vi "Create_Error_log_folders.vi"(0 "Log Filename":string, 1 "Days ago":dbl, 2 "Log Folder":string, 3 "Per Day Log File?":bool) -> (5 "Local Log File":path, 7 "exists?":bool)   [LabVIEW 2022 SP3]
uses:
  Globals/Preference_global.vi
  Globals/Constants_global.vi
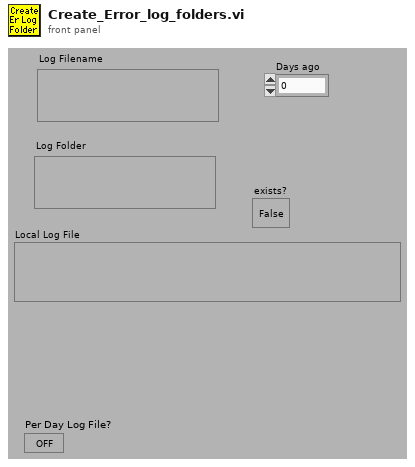
[diagram p1: front panel]
types:
  T1 = cluster{"second":i32, "minute":i32, "hour":i32, "day of month":i32, "month":i32, "year":i32, "day of week":i32, "day of year":i32, "is DST":i32}
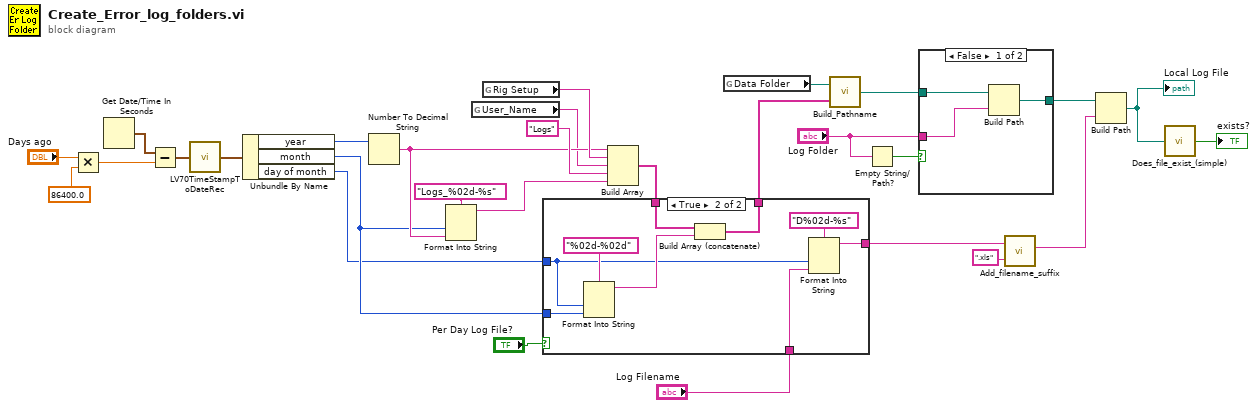
[diagram p0: block diagram]
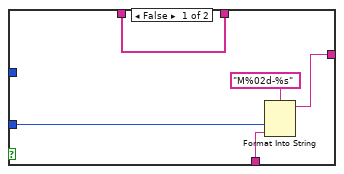
[diagram p2: hidden frame]
diagram:
  n1 = Multiply(x="Days ago", y=86400.0) -> (x*y=w2:dbl)
  n2 = Get Date/Time In Seconds() -> (seconds since 1Jan1904=w5:timestamp)
  n3 = Subtract(x=w5, y=w2) -> (x-y=w1:timestamp)
  n4 = call <vilib>:"LV70TimeStampToDateRec.vi"("time stamp"=w1) -> ("date time rec"=w29:T1)
  n5 = Unbundle By Name(w29) -> ("year"=w28:i32, "month"=w9:i32, "day of month"=w8:i32)
  n6 = Number To Decimal String(number=w28) -> (decimal integer string=w22:string)  [unwired: 1 out]
  n7 = Format Into String(format string="Logs_%02d-%s", w9, w22) -> (resulting string=w20:string)  [unwired: 2 in, 1 out]
  n8 = global read "Preference_global.vi" "User_Name"() -> (w11:string)
  n9 = global read "Preference_global.vi" "Rig Setup"() -> (w24:string)
  n10 = Build Array(w22, w24, w11, "Logs", w20) -> (w13:string[])
  n11 = case shown="True" "Per Day Log File?" {
    tunnel: w8 -> [_ w35]
    tunnel: w13 -> [w34 w41]
    tunnel: [w34 w40] -> w12
    tunnel: w9 -> [w30 w39]
    tunnel: "Log Filename" -> [w32 w37]
    tunnel: [w31 w36] -> w6
    frame False {
      n12 = Format Into String(format string="M%02d-%s", w30, w32) -> (resulting string=w31:string)  [unwired: 2 in, 1 out]
    }
    frame True {
      n13 = Format Into String(format string="%02d-%02d", w35, w39) -> (resulting string=w42:string)  [unwired: 2 in, 1 out]
      n14 = Build Array (concatenate)(w41, w42) -> (w40:string[])
      n15 = Format Into String(format string="D%02d-%s", w35, w37) -> (resulting string=w36:string)  [unwired: 2 in, 1 out]
    }
  }
  n16 = global read "Constants_global.vi" "Data Folder"() -> (w18:path)
  n17 = call "Build_Pathname.vi"("PathElements"=w12, "PathnameIn"=w18) -> ("AppendedPath"=w17:path)
  n18 = Empty String/Path?(string/path="Log Folder") -> (empty?=w25:bool)
  n19 = case shown="False" w25 {
    tunnel: "Log Folder" -> [w45 _]
    tunnel: w17 -> [w46 w47]
    tunnel: [w44 w47] -> w16
    frame False {
      n20 = Build Path(base path=w46, name or relative path=w45) -> (appended path=w44:path)
    }
    frame True {
    }
  }
  n21 = call "Add_filename_suffix.vi"("Filename"=w6, "Suffix to add"=".xls") -> ("Filename out"=w15:string)  [unwired: 3 out]
  n22 = Build Path(base path=w16, name or relative path=w15) -> (appended path=w10:path)
  "Local Log File" <- w10
  n23 = call "Does_file_exist_(simple).vi"("Pathname"=w10) -> ("exists?"=→"exists?":bool)
